vi "FTW-Crypto-String-Sign.vi"(0 "String":string, 5 "Private Signing Key":string, 7 "Regex to Match Signature":string="\"Signature\"(?:\\s*)?:(?:\\s*)?\"\\K(.*?)(?=\")", 11 "error in":errorcluster) -> (4 "Signed String":string, 6 "Signed Successfully":bool, 8 "Valid Signing Key Structure":bool, 15 "error out":errorcluster)   [LabVIEW 2015]
panel:
  # "Inputs"
  # "Outputs"
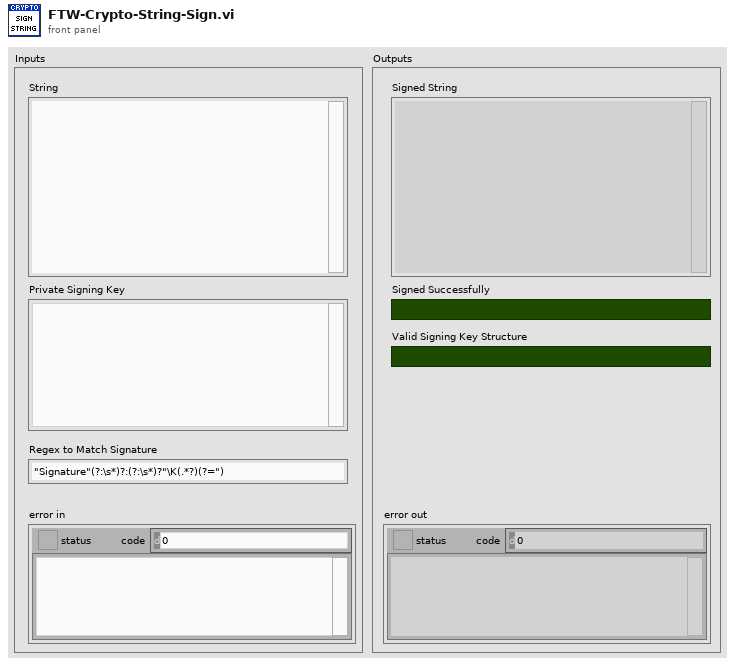
[diagram p1: front panel]
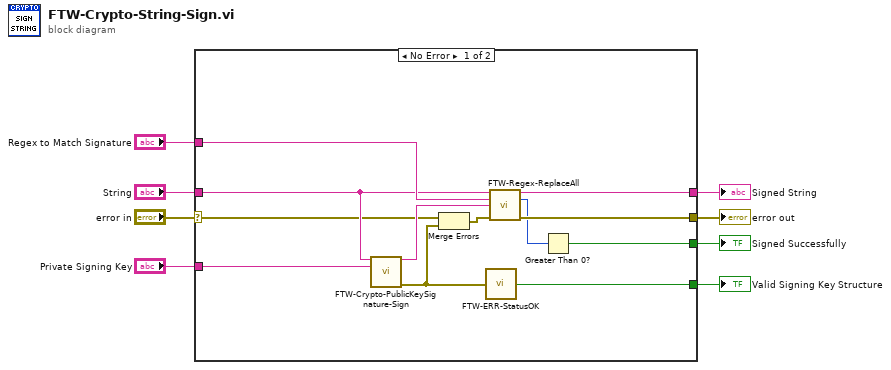
[diagram p0: block diagram]
diagram:
  n1 = case shown="No Error" "error in" {
    selector: "error in" -> [w13 w22]
    tunnel: [w14 w22] -> w8
    tunnel: "String" -> [w17 w21]
    tunnel: [w16 w21] -> w5
    tunnel: "Private Signing Key" -> [w20 _]
    tunnel: "Regex to Match Signature" -> [w18 _]
    tunnel: [w19 _] -> w2
    tunnel: [w9 _] -> w1
    frame No Error {
      n2 = call "FTW-Crypto-PublicKeySignature-Sign.vi"("Data"=w17, "Private Key XML"=w20) -> ("Hex Encoded Signature"=w15:string, "error out"=w12:errorcluster)  [unwired: 11 in, 1 out]
      n3 = Merge Errors(w13, w12) -> (w11:errorcluster)
      n4 = call "FTW-ERR-StatusOK.vi"("error to check"=w12) -> ("Status OK?"=w19:bool)
      n5 = call "FTW-Regex-ReplaceAll.vi"("String"=w17, "Search for (Regular Expression)"=w18, "Replace with"=w15, "error in"=w11) -> ("String out"=w16:string, "Number of Replacements"=w10:i32, "error out"=w14:errorcluster)  [unwired: 9 in]
      n6 = Greater Than 0?(x=w10) -> (x > 0?=w9:bool)
    }
    frame Error {
    }
  }
  "error out" <- w8
  "Signed String" <- w5
  "Valid Signing Key Structure" <- w2
  "Signed Successfully" <- w1
